vi "Init.vi"(8 "error in":errorcluster) -> (0 "error out":errorcluster, 3 "Match out":refnum<class "Match.lvclass">)   [LabVIEW 2016, in "Match.lvclass"]
uses:
  Match.lvclass
  Match.lvclass/Match.ctl
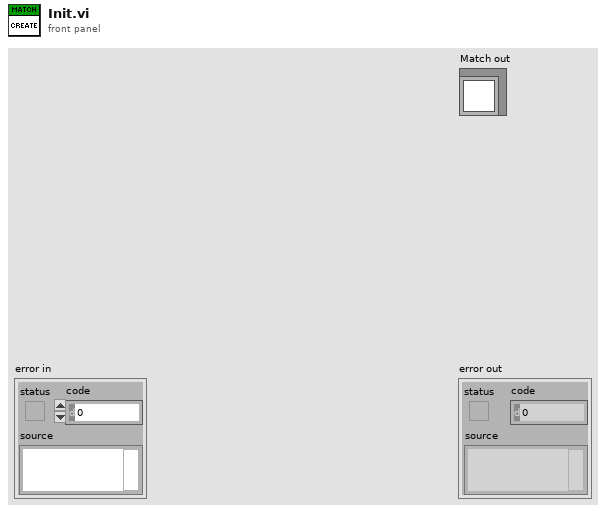
[diagram p1: front panel]
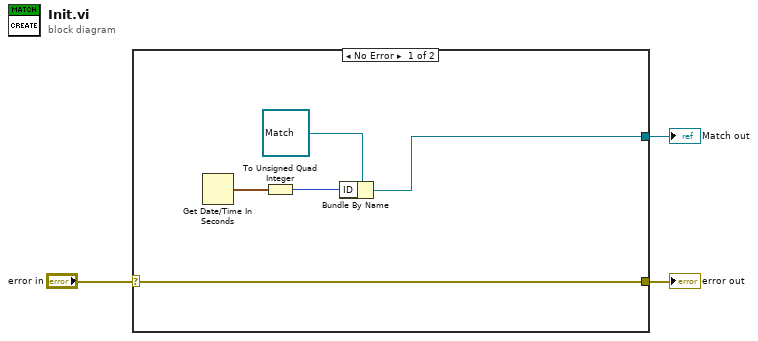
[diagram p0: block diagram]
diagram:
  n1 = case shown="No Error" "error in" {
    selector: "error in" -> [w8 w9]
    tunnel: [w8 w9] -> w2
    tunnel: [w7 _] -> w1
    frame No Error {
      n2 = Get Date/Time In Seconds() -> (seconds since 1Jan1904=w5:timestamp)
      n3 = To Unsigned Quad Integer(1:w5) -> (0:w4:u64)
      n4 = Bundle By Name(cluster=refnum<class "Match.lvclass"> refnum ("Match in"), "ID"=w4) -> (w7:refnum<class "Match.lvclass">)
    }
    frame Error {
    }
  }
  "error out" <- w2
  "Match out" <- w1
